vi "Write Time Stamp.vi"(8 "error in (no error)":errorcluster, 10 "Time Stamp":timestamp, 11 "TDMS-Data in":refnum<class "TDMS-Data.lvclass">) -> (0 "error out":errorcluster, 3 "TDMS-Data out":refnum<class "TDMS-Data.lvclass">)   [LabVIEW 2014, in "BNT_TDMS.lvlib" / "TDMS-Data.lvclass"]
doc: "Write timestamp attribute."
uses:
  TDMS-Data.lvclass
  TDMS-Data.lvclass/TDMS-Data.ctl
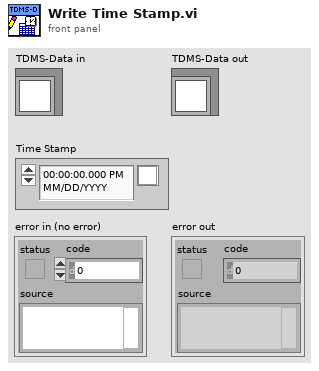
[diagram p1: front panel]
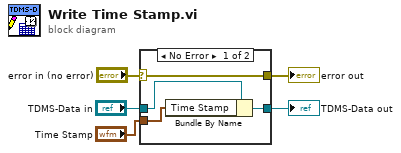
[diagram p0: block diagram]
diagram:
  n1 = case shown="No Error" "error in (no error)" {
    selector: "error in (no error)" -> [w9 w10]
    tunnel: [w9 w10] -> w4
    tunnel: [w7 w11] -> w2
    tunnel: "TDMS-Data in" -> [w8 w11]
    tunnel: "Time Stamp" -> [w6 _]
    frame No Error {
      n2 = Bundle By Name(cluster=w8, "Time Stamp"=w6) -> (w7:refnum<class "TDMS-Data.lvclass">)
    }
    frame Error {
    }
  }
  "error out" <- w4
  "TDMS-Data out" <- w2
